vi "AddNewNode.vi"(7 "Attributes":string[][](array[string]), 8 "Insert As Child":bool, 9 "New Node Name":string, 10 "Node ID":string, 11 "DOM document":refnum<k20>) -> ()   [LabVIEW 2017]
uses:
  <vilib>/xml/NI_XML.lvlib
  <resource>/objmgr/DOMUserDefRef.rc
panel:
  out "appended array":string[][](array[string])
  out "XML":string
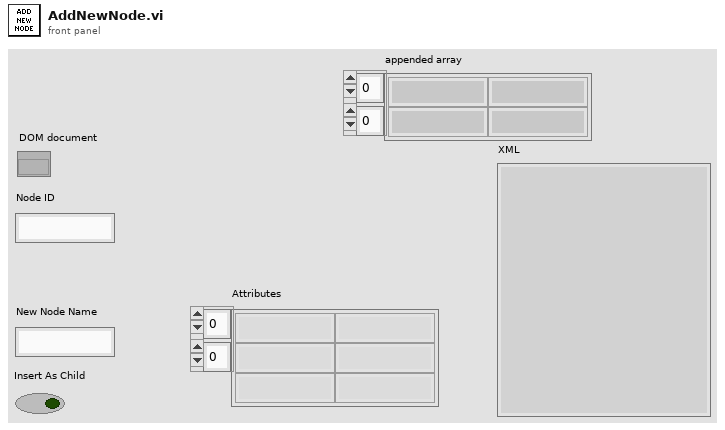
[diagram p1: front panel]
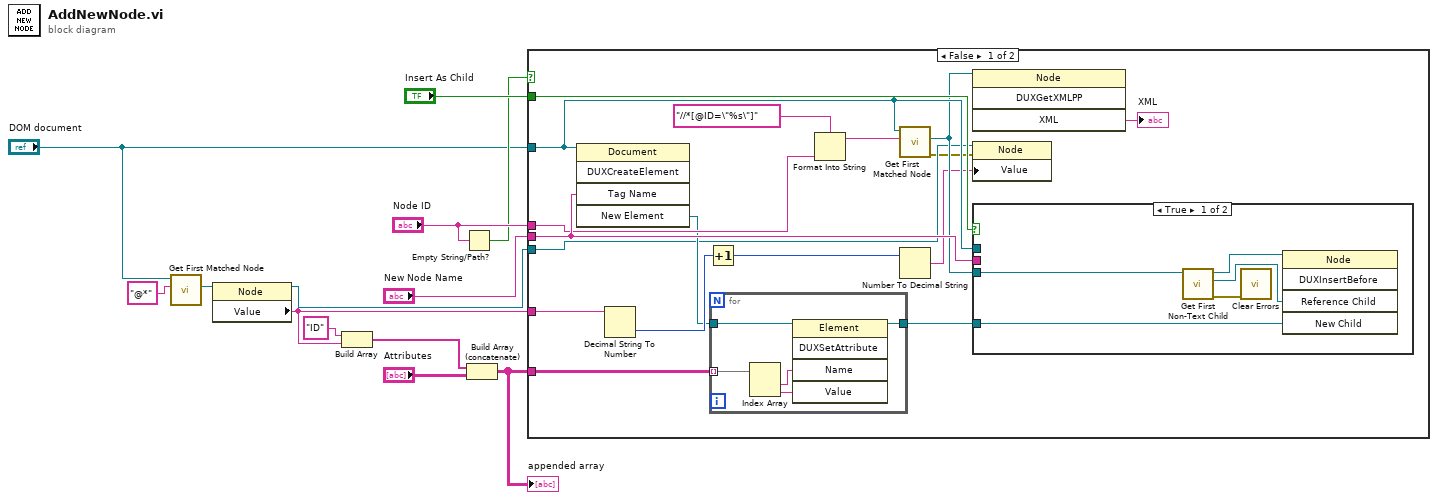
[diagram p0: block diagram]
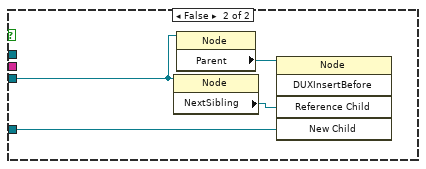
[diagram p2: hidden frame]
diagram:
  n1 = call <vilib>:"Get First Matched Node.vi"("XPath expression"="@*", "node in"="DOM document") -> ("node result"=w7:refnum<k20>)  [unwired: 7 in, 2 out]
  n2 = property class="Node"(reference=w7) -> (reference out=w5:refnum<k20>, "Value"=w2:string)  [unwired: 1 in, 1 out]
  n3 = Build Array("ID" ("XPath expression"), w2) -> (w8:string[])
  n4 = Empty String/Path?(string/path="Node ID") -> (empty?=w10:bool)
  n5 = Build Array (concatenate)(w8, "Attributes") -> (w1:string[][])
  "appended array" <- w1
  n6 = case shown="False" w10 {
    tunnel: "DOM document" -> [w30 _]
    tunnel: "Insert As Child" -> [w29 _]
    tunnel: "New Node Name" -> [w28 _]
    tunnel: "Node ID" -> [w20 _]
    tunnel: w5 -> [w17 _]
    tunnel: w2 -> [w16 _]
    tunnel: w1 -> [w15 _]
    frame False {
      n7 = invoke class="Document" method="DUXCreateElement"(reference=w30, "Tag Name"=w28) -> ("New Element"=w19:refnum<k20>)  [unwired: 3 in, 4 out]
      n8 = Decimal String To Number(string=w16) -> (number=w21:i32)  [unwired: 2 in, 1 out]
      n9 = Increment(x=w21) -> (x+1=w22:i32)
      n10 = for {
        tunnel: w19 -> [w35]
        tunnel: [w34] -> w18
        tunnel: w15 -> [w33] mode=indexing
        n11 = Index Array(array=w33) -> (element #1=w32:string, element #2=w31:string)  [unwired: 2 in]
        n12 = invoke class="Element" method="DUXSetAttribute"(reference=w35, "Name"=w32, "Value"=w31) -> (reference out=w34:refnum<k20>)  [unwired: 2 in, 4 out]
      }
      n13 = Format Into String(format string="//*[@ID=\"%s\"]", w20) -> (resulting string=w24:string)  [unwired: 2 in, 1 out]
      n14 = call <vilib>:"Get First Matched Node.vi"("XPath expression"=w24, "node in"=w30) -> ("error out"=w14:errorcluster, "node result"=w26:refnum<k20>)  [unwired: 7 in, 1 out]
      n15 = Number To Decimal String(number=w22) -> (decimal integer string=w23:string)  [unwired: 1 in]
      n16 = invoke class="Node" method="DUXGetXMLPP"(reference=w26) -> ("XML"=→"XML":string)  [unwired: 3 in, 3 out]
      n17 = property class="Node"(reference=w17, error in=w14, "Value"=w23) -> ()  [unwired: 2 out]
      n18 = case shown="True" w29 {
        tunnel: w30 -> [_ _]
        tunnel: w28 -> [_ _]
        tunnel: w26 -> [w37 w43]
        tunnel: w18 -> [w36 w41]
        frame True {
          n19 = call <vilib>:"Get First Non-Text Child.vi"("node in"=w37) -> ("error out"=w38:errorcluster, "child node"=w39:refnum<k20>, "node out"=w40:refnum<k20>)  [unwired: 7 in, 1 out]
          n20 = call <vilib>:"Clear Errors.vi"("error in (no error)"=w38) -> ()  [unwired: 5 in, 2 out]
          n21 = invoke class="Node" method="DUXInsertBefore"(reference=w40, "Reference Child"=w39, "New Child"=w36) -> ()  [unwired: 2 in, 5 out]
        }
        frame False {
          n22 = property class="Node"(reference=w43) -> ("NextSibling"=w44:refnum<k20>)  [unwired: 1 in, 2 out]
          n23 = property class="Node"(reference=w43) -> ("Parent"=w42:refnum<k20>)  [unwired: 1 in, 2 out]
          n24 = invoke class="Node" method="DUXInsertBefore"(reference=w42, "Reference Child"=w44, "New Child"=w41) -> ()  [unwired: 2 in, 5 out]
        }
      }
    }
    frame True {
      # "Not a valid selection,\ndon't add any nodes"
    }
  }
